vi "Washers Diameters.vi"() -> ()   [LabVIEW 2020]
uses:
  <vilib>/Analysis/NI_AALBase.lvlib
panel:
  out "Deviazione standard":dbl format="%0.2f"
  out "Spessore medio":dbl format="%0.2f"
  out "error out":errorcluster
  out "Diametro esterno":dbl[](array[numeric])
  out "Diametro interno":dbl[](array[numeric])
  in  "Calibration Image":path=path "C:/Users/Dell/Documents/Vision-System/Images/CalibGrid_10mm.png"
  out "Image":T1(plugin-control)
  in  "error in (no error)":errorcluster
  in  "Image Path":path=path "C:/Users/Dell/Documents/Vision-System/Images/washers.jpg"
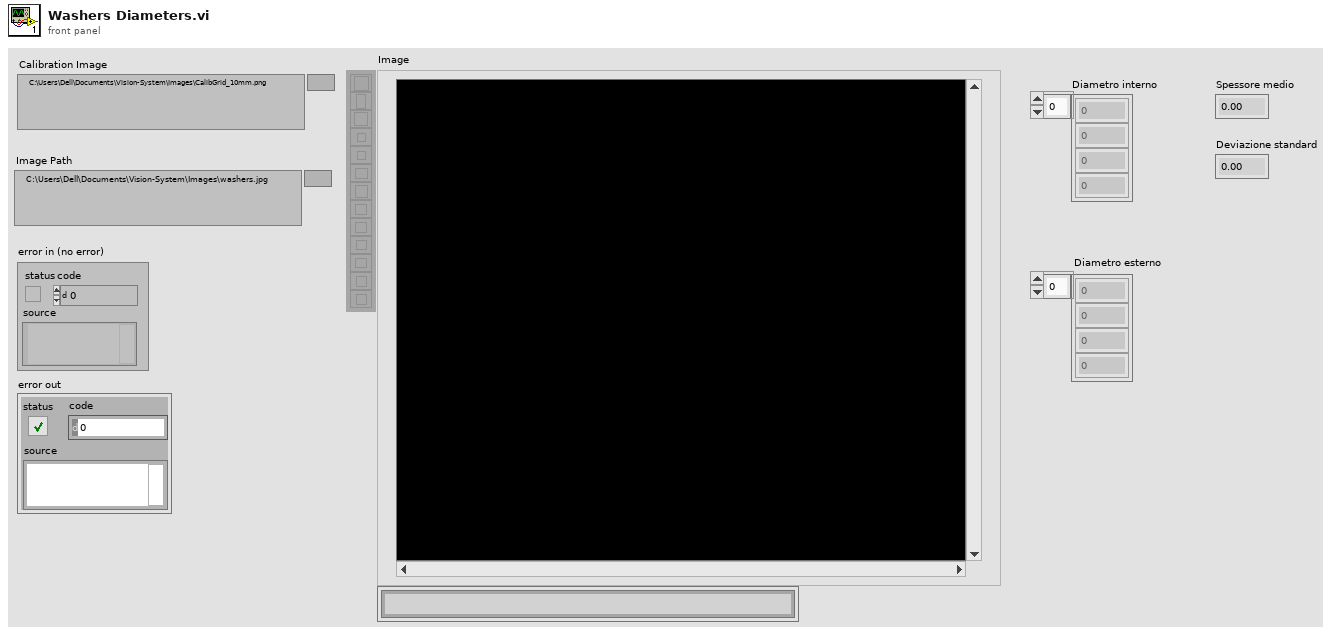
[diagram p1: front panel]
types:
  T1 = typedef "IMAQ Image.ctl" = refnum<image>
  T2 = typedef "Edge New.ctl" = cluster{"Location (Pixel)":cluster{"X":sgl, "Y":sgl}, "Location (Real-World)":cluster{"X":sgl, "Y":sgl}, "Distance (Pixel)":dbl, "Distance (Real-World)":dbl, "Strength":dbl, "Noise":dbl, "Rising?":bool}
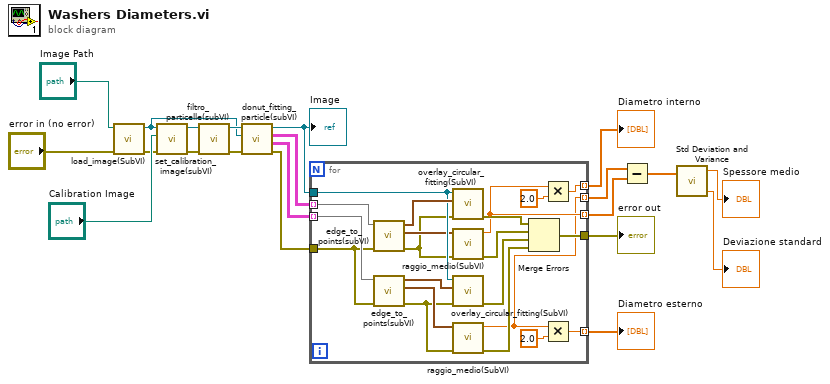
[diagram p0: block diagram]
diagram:
  n1 = call "load_image(SubVI).vi"("error in (no error)"="error in (no error)", "Image Path"="Image Path") -> ("error out"=w13:errorcluster, "Image GRAY"=w9:T1)  [unwired: 8 in]
  n2 = call "set_calibration_image(subVI).vi"("error in (no error)"=w13, "File Path"="Calibration Image", "Image Dst"=w9) -> ("error out"=w14:errorcluster, "Image Out"=w15:T1)  [unwired: 6 in, 1 out]
  n3 = call "filtro_particelle(subVI).vi"("error in (no error)"=w14, "Image Src"=w15) -> ("error out"=w18:errorcluster, "Image"=w19:T1)  [unwired: 8 in]
  n4 = call "donut_fitting_particle(subVI).vi"("error in (no error)"=w18, "Image Dst"=w9, "Image Src"=w19) -> ("error out"=w11:errorcluster, "First Edges"=w12:T2[][], "Last Edges"=w17:T2[][], "Image"=w10:T1)  [unwired: 5 in]
  "Image" <- w10
  n5 = for {
    tunnel: w17 -> [w42] mode=indexing
    tunnel: w12 -> [w41] mode=indexing
    tunnel: w11 -> [w40]
    tunnel: w10 -> [w38]
    tunnel: [w24] -> w3 mode=indexing
    tunnel: [w26] -> w4 mode=indexing
    tunnel: [w28] -> w8
    tunnel: [w23] -> w2 mode=indexing
    tunnel: [w22] -> w1 mode=indexing
    n6 = call "edge_to_points(subVI).vi"("error in (no error)"=w40, "First Edges"=w42) -> ("error out"=w34:errorcluster, "points (real-world)"=w36:cluster{"X":sgl, "Y":sgl}[], "points (pixel)"=w39:cluster{"X":sgl, "Y":sgl}[])  [unwired: 7 in]
    n7 = call "edge_to_points(subVI).vi"("error in (no error)"=w40, "First Edges"=w41) -> ("error out"=w33:errorcluster, "points (real-world)"=w35:cluster{"X":sgl, "Y":sgl}[], "points (pixel)"=w37:cluster{"X":sgl, "Y":sgl}[])  [unwired: 7 in]
    n8 = call "overlay_circular_fitting(SubVI).vi"("error in (no error)"=w34, "points (pixel)"=w39, "image dest"=w38) -> ("error out"=w32:errorcluster)  [unwired: 6 in, 2 out]
    n9 = call "raggio_medio(SubVI).vi"("error in (no error)"=w34, "Radial Points"=w36) -> ("error out"=w31:errorcluster, "Radius"=w23:dbl)  [unwired: 8 in]
    n10 = call "overlay_circular_fitting(SubVI).vi"("error in (no error)"=w33, "points (pixel)"=w37, "image dest"=w38) -> ("error out"=w30:errorcluster)  [unwired: 6 in, 2 out]
    n11 = call "raggio_medio(SubVI).vi"("error in (no error)"=w33, "Radial Points"=w35) -> ("error out"=w29:errorcluster, "Radius"=w22:dbl)  [unwired: 8 in]
    n12 = Merge Errors(w32, w31, w30, w29) -> (w28:errorcluster)
    n13 = Multiply(x=w23, y=2.0) -> (x*y=w24:dbl)
    n14 = Multiply(x=w22, y=2.0) -> (x*y=w26:dbl)
  }
  "Diametro interno" <- w3
  "Diametro esterno" <- w4
  "error out" <- w8
  n15 = Subtract(x=w1, y=w2) -> (x-y=w5:dbl[])
  n16 = call <vilib>:"Std Deviation and Variance.vi"("X"=w5) -> ("mean"=→"Spessore medio":dbl, "variance"=→"Deviazione standard":dbl)  [unwired: 1 in, 1 out]
